vi "Select ini file GUI.vi"(4 "Command":enum16{"Initialize", "Update"}(ring)=enum."Update", 5 "ok":refnum<vi>, 6 "Delete Instance":refnum<vi>, 7 "Instances":refnum<vi>, 8 "error in (no error)":errorcluster, 9 "Device":refnum<vi>, 10 "Device control":refnum<vi>, 11 "Select":refnum<vi>) -> (0 "error out":errorcluster, 3 "Name":string)   [LabVIEW 2015]
uses:
  Instance.ctl
  Calibration and Function folders.ctl
  file/file action.ctl
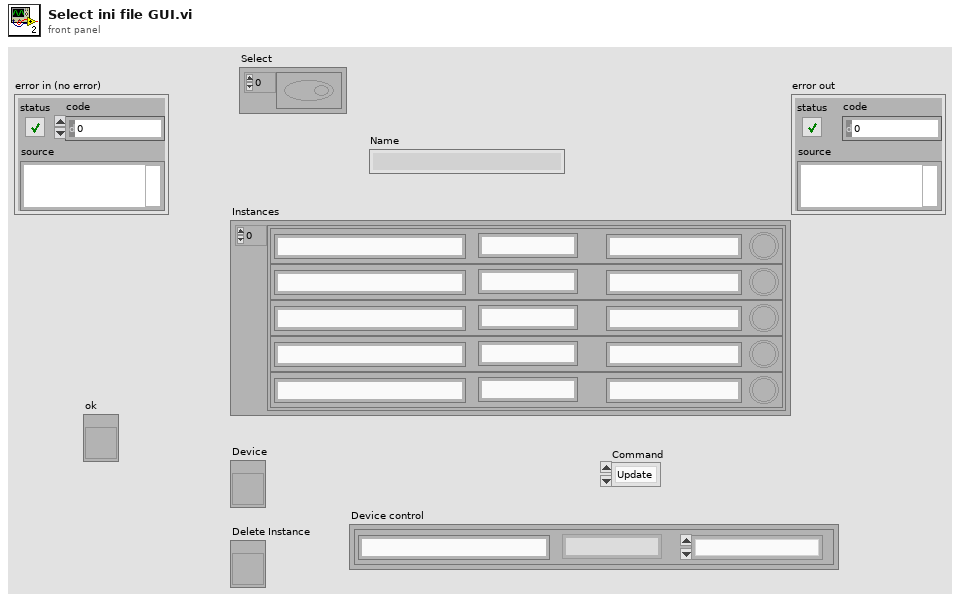
[diagram p1: front panel]
types:
  T1 = typedef "Calibration and Function folders.ctl" = enum16{"Sensors", "Functions", "Config File", "PublicAppFolder", "New ini File", "Set Config File", "Delete ini File"}
  T2 = typedef "file action.ctl" = enum16{"Save", "Open"}
  T3 = typedef "Instance.ctl" = cluster{"Name":string, "Device Name":string, "Running":bool, "File Name":string}
  T4 = cluster{"Name":string, "File Name":string, "Device":u16}
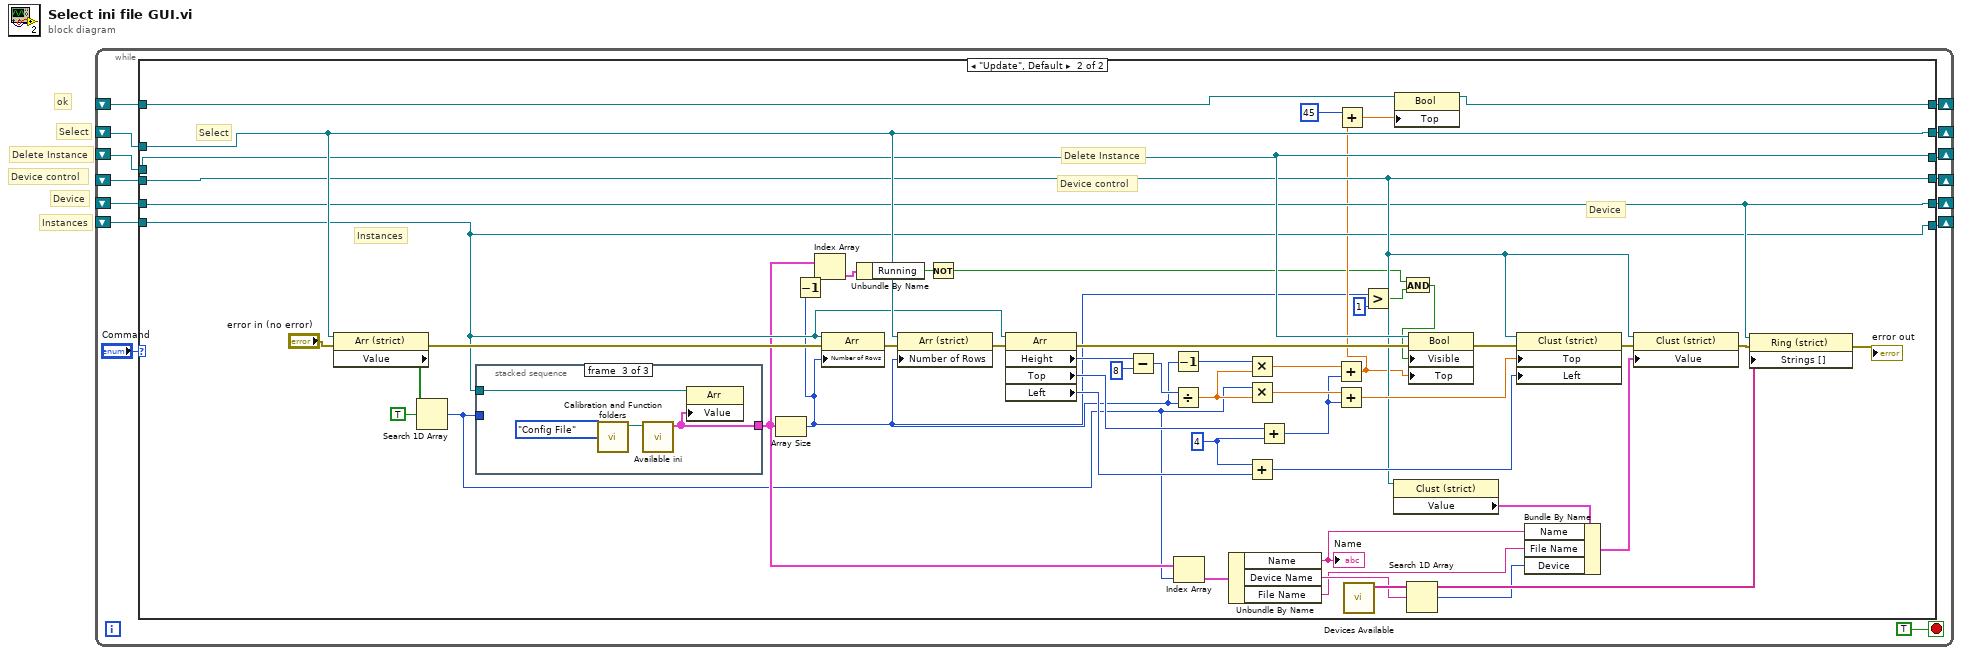
[diagram p0: block diagram]
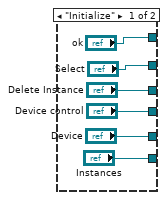
[diagram p2: hidden frame]
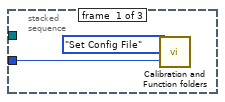
[diagram p3: hidden frame]
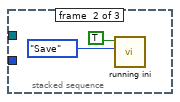
[diagram p4: hidden frame]
diagram:
  # "ok"
  # "Instances"
  # "Device"
  # "Device control"
  # "Delete Instance"
  # "Select"
  n1 = while {
    shift-right: [w14] -> _
    shift-left: _ -> [w9]
    shift-right: [w13] -> _
    shift-left: _ -> [w8]
    shift-right: [w12] -> _
    shift-left: _ -> [w7]
    shift-right: [w11] -> _
    shift-left: _ -> [w6]
    shift-right: [w10] -> _
    shift-left: _ -> [w5]
    shift-right: [w2] -> _
    shift-left: _ -> [w1]
    stop <- TRUE stop-if-true
    n2 = case shown="\"Update\", Default" "Command" {
      tunnel: ["Select" w40] -> w14
      tunnel: ["Delete Instance" w39] -> w13
      tunnel: ["Device control" w38] -> w12
      tunnel: ["Device" w37] -> w11
      tunnel: ["Instances" w36] -> w10
      tunnel: w9 -> [_ w40]
      tunnel: w8 -> [_ w39]
      tunnel: w7 -> [_ w38]
      tunnel: w6 -> [_ w37]
      tunnel: w5 -> [_ w36]
      tunnel: ["ok" w34] -> w2
      tunnel: w1 -> [_ w35]
      frame "Initialize" {
      }
      frame "Update", Default {
        w53 = 4 ("x")
        # "Select"
        # "Instances"
        # "Delete Instance"
        # "Device control"
        # "Device"
        n3 = property on="Property Node" class="Arr (strict)"(reference=w40, error in="error in (no error)") -> (error out=w68:errorcluster, "Value"=w61:bool[])  [unwired: 1 out]
        n4 = Search 1D Array(1D array=w61, element=TRUE) -> (index of element=w28:i32)  [unwired: 1 in]
        n5 = stacked-sequence {
          tunnel: w28 -> [w73 _ _]
          tunnel: [_ _ w78] -> w29
          tunnel: w36 -> [_ _ w77]
          frame #0 {
            n6 = call "Calibration and Function folders.vi"("ini file index"=w73, "Folder"=Calibration_and_Function_folders."Set Config File") -> ()  [unwired: 8 in, 2 out]
          }
          frame #1 {
            n7 = call "running ini.vi"("running in"=TRUE ("running"), "Action"=file_action."Save") -> ()  [unwired: 4 in, 1 out]
          }
          frame #2 {
            n8 = call "Calibration and Function folders.vi"("Folder"=Calibration_and_Function_folders."Config File") -> ("Selected Folder"=w79:path)  [unwired: 9 in, 1 out]
            n9 = call "Available ini.vi"("Config file path"=w79) -> ("Instances"=w78:T3[])  [unwired: 5 in, 5 out]
            n10 = property class="Arr"(reference=w77, "Value"=w78) -> ()  [unwired: 1 in, 2 out]
          }
        }
        n11 = Array Size(array=w29) -> (size(s)=w22:i32)
        n12 = Decrement(x=w22) -> (x-1=w21:i32)
        n13 = Index Array(array=w29, index=w21) -> (element=w27:T3)
        n14 = property on="Property Node" class="Arr"(reference=w36, error in=w68, "Number of Rows"=w22) -> (error out=w65:errorcluster)  [unwired: 1 out]
        n15 = Unbundle By Name(w27) -> ("Running"=w26:bool)
        n16 = property on="Property Node" class="Arr (strict)"(reference=w40, error in=w65, "Number of Rows"=w22) -> (error out=w69:errorcluster)  [unwired: 1 out]
        n17 = Not(x=w26) -> (.not. x?=w24:bool)
        n18 = property on="Property Node" class="Arr"(reference=w36, error in=w69) -> (error out=w62:errorcluster, "Height"=w55:u32, "Top"=w43:i32, "Left"=w42:i32)  [unwired: 1 out]
        n19 = Subtract(x=w55, y=u32 8) -> (x-y=w56:u32)
        n20 = Decrement(x=w22) -> (x-1=w70:i32)
        n21 = Divide(x=w56, y=w22) -> (x/y=w45:dbl)
        n22 = Index Array(array=w29, index=w28) -> (element=w59:T3)
        n23 = Unbundle By Name(w59) -> ("Name"=w41:string, "Device Name"=w58:string, "File Name"=w49:string)
        "Name" <- w41
        n24 = Multiply(x=w70, y=w45) -> (x*y=w44:dbl)
        n25 = Multiply(x=w28, y=w45) -> (x*y=w57:dbl)
        n26 = Add(x=w53, y=w42) -> (x+y=w48:i32)
        n27 = Add(x=w43, y=w53) -> (x+y=w46:i32)
        n28 = Add(x=w44, y=w46) -> (x+y=w31:dbl)
        n29 = Add(x=w57, y=w46) -> (x+y=w47:dbl)
        n30 = Add(x=45 ("Position:Top"), y=w31) -> (x+y=w32:dbl)
        n31 = call "Devices Available.vi"() -> ("Devices"=w67:string[])  [unwired: 7 in, 4 out]
        n32 = Greater?(x=w22, y=1 ("x")) -> (0:w25:bool)
        n33 = property class="Clust (strict)"(reference=w38) -> ("Value"=w52:T4)  [unwired: 1 in, 2 out]
        n34 = property class="Bool"(reference=w35, "Top"=w32) -> (reference out=w34:refnum<vi>)  [unwired: 1 in, 1 out]
        n35 = And(x=w24, y=w25) -> (x .and. y?=w23:bool)
        n36 = Search 1D Array(1D array=w67, element=w58) -> (index of element=w50:i32)  [unwired: 1 in]
        n37 = property on="Property Node" class="Bool"(reference=w39, error in=w62, "Visible"=w23, "Top"=w31) -> (error out=w63:errorcluster)  [unwired: 1 out]
        n38 = property on="Property Node" class="Clust (strict)"(reference=w38, error in=w63, "Top"=w47, "Left"=w48) -> (error out=w64:errorcluster)  [unwired: 1 out]
        n39 = Bundle By Name(cluster=w52, "Name"=w41, "File Name"=w49, "Device"=w50) -> (w51:T4)
        n40 = property class="Clust (strict)"(reference=w38, error in=w64, "Value"=w51) -> (error out=w71:errorcluster)  [unwired: 1 out]
        n41 = property on="Property Node" class="Ring (strict)"(reference=w37, error in=w71, "Strings []"=w67) -> (error out=→"error out":errorcluster)  [unwired: 1 out]
      }
    }
  }
